vi "test-dataPreview.vi"(8 "error in (no error)":errorcluster, 11 "TestCase in":refnum<class "MyTestCase.lvclass">) -> (0 "error out":errorcluster, 3 "TestCase out":refnum<class "MyTestCase.lvclass">)   [LabVIEW 2019, in "MyTestCase.lvclass"]
uses:
  MyTestCase.lvclass
  <vilib>/addons/_JKI Toolkits/VI Tester/TestCase.llb/TestCase.lvclass
  C:/Program Files (x86)/National Instruments/LabVIEW 2019/vi.lib/addons/_JKI Toolkits/VI Tester/TestCase.llb/TestCase.lvclass
panel:
  in  "Tree 2":string(tree)
  in  "Tree":string(tree)
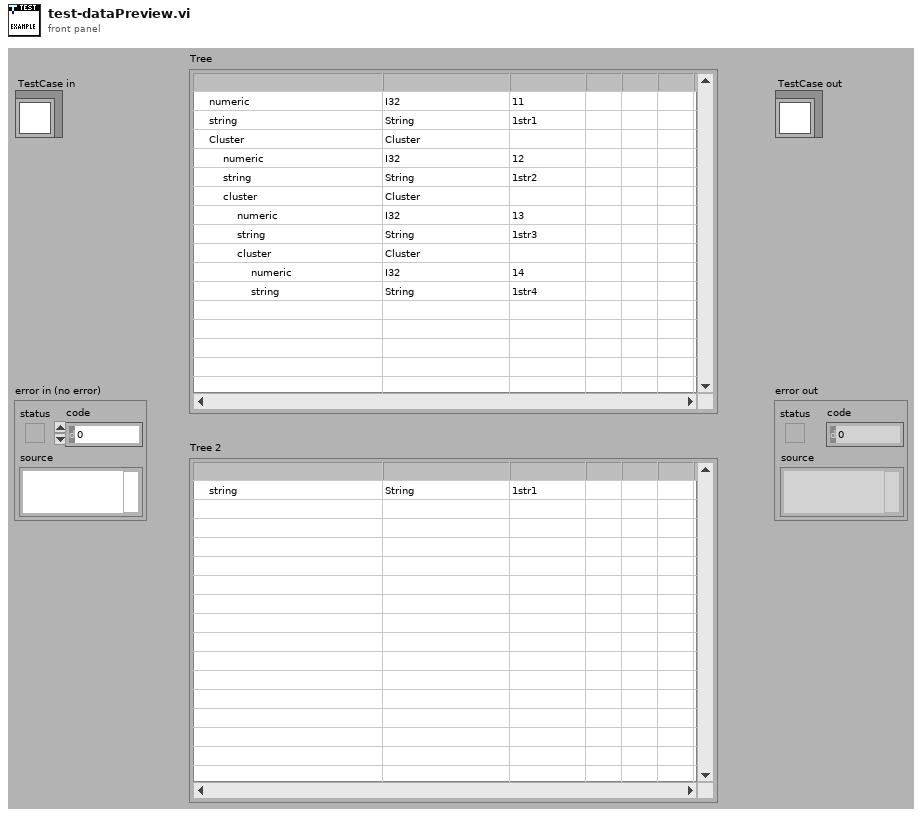
[diagram p1: front panel]
types:
  T1 = cluster{"numeric":i32, "string":string, "Cluster":cluster{"numeric":i32, "string":string, "cluster":cluster{"numeric":i32, "string":string, "cluster":cluster{"numeric":i32, "string":string}}}}
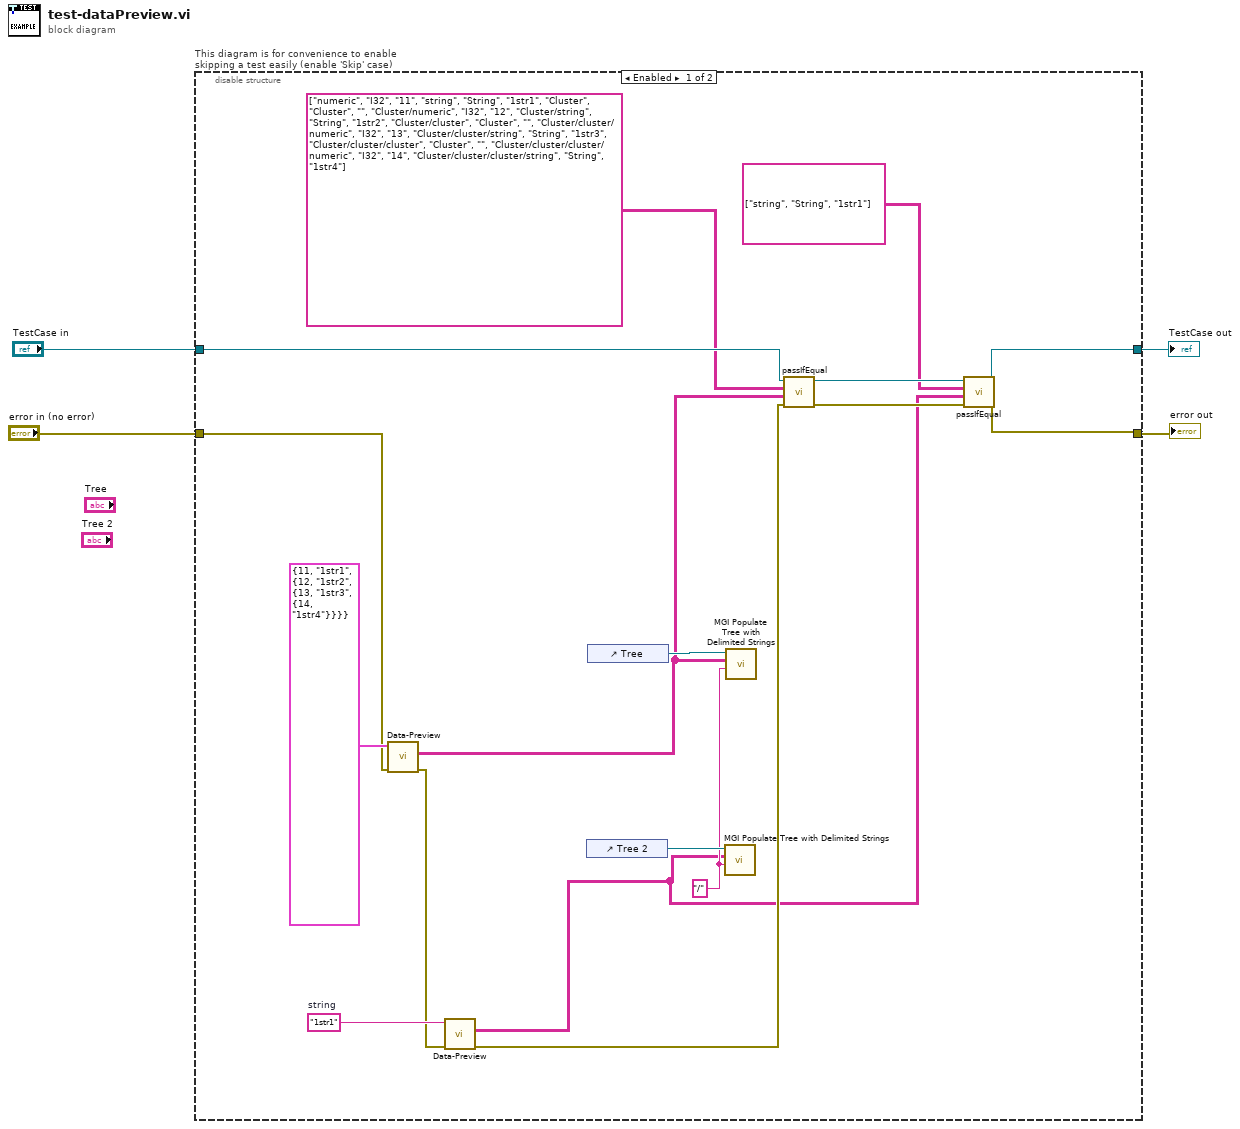
[diagram p0: block diagram]
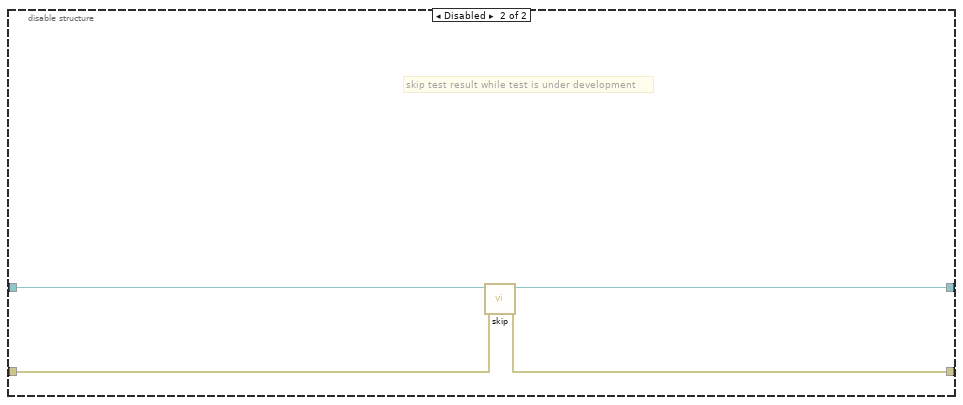
[diagram p2: hidden frame]
diagram:
  n1 = disable-structure "This diagram is for convenience to enable skipping a test easily (enable 'Skip' case)" shown="Enabled" {
    disable-tunnel: "TestCase in" -> [w12 w25]
    disable-tunnel: [w21 w23] -> w1
    disable-tunnel: [w20 w24] -> w3
    disable-tunnel: "error in (no error)" -> [w13 w22]
    frame Enabled {
      w17 = "1str1"  # string
      w15 = "/" ("Delimiter")
      n2 = call "Data-Preview.vi"("error in"=w13, "data"=T1 {"numeric"=11, "string"="1str1", "Cluster"={"numeric"=12, "string"="1str2", "cluster"={"numeric"=13, "string"="1str3", "cluster"={"numeric"=14, "string"="1str4"}}}} ("Cluster")) -> ("error out"=w14:errorcluster, "Array"=w7:string[][])  [unwired: 7 in, 1 out]
      n3 = call "Data-Preview.vi"("error in"=w14, "data"=w17) -> ("error out"=w9:errorcluster, "Array"=w5:string[][])  [unwired: 7 in, 1 out]
      n4 = control-ref of="Tree 2"() -> (w16:refnum<vi>)
      n5 = control-ref of="Tree"() -> (w18:refnum<vi>)
      n6 = call <userlib>:"MGI Populate Tree with Delimited Strings.vi"("Delimiter"=w15, "Items (Delimited)"=w5, "Tree Control"=w16) -> ()  [unwired: 6 in, 3 out]
      n7 = call <userlib>:"MGI Populate Tree with Delimited Strings.vi"("Delimiter"=w15, "Items (Delimited)"=w7, "Tree Control"=w18) -> ()  [unwired: 6 in, 3 out]
      n8 = call-dynamic "passIfEqual.vi"("error in (no error)"=w9, "y"=w7, "x"=string[][] [["numeric", "I32", "11"], ["string", "String", "1str1"], ["Cluster", "Cluster", ""], ["Cluster/numeric", "I32", "12"], ["Cluster/string", "String", "1str2"], ["Cluster/cluster", "Cluster", ""], ["Cluster/cluster/numeric", "I32", "13"], ["Cluster/cluster/string", "String", "1str3"], ["Cluster/cluster/cluster", "Cluster", ""], ["Cluster/cluster/cluster/numeric", "I32", "14"], ["Cluster/cluster/cluster/string", "String", "1str4"]] ("Array 2"), "TestCase in"=w12) -> ("error out"=w10:errorcluster, "TestCase out"=w11:refnum<class "MyTestCase.lvclass">)  [unwired: 6 in]
      n9 = call-dynamic "passIfEqual.vi"("error in (no error)"=w10, "y"=w5, "x"=string[][] [["string", "String", "1str1"]] ("Array"), "TestCase in"=w11) -> ("error out"=w20:errorcluster, "TestCase out"=w21:refnum<class "MyTestCase.lvclass">)  [unwired: 6 in]
    }
    frame Disabled {
      # "skip test result while test is under development"
      n10 = call <vilib>:"skip.vi"("error in (no error)"=w22, "TestCase in"=w25) -> ("error out"=w24:errorcluster, "TestCase out"=w23:refnum<class "MyTestCase.lvclass">)  [unwired: 8 in]
    }
  }
  "error out" <- w3
  "TestCase out" <- w1
